vi "FT10_FPGA_7854R_Main 4.vi"(8 "Conn2 DIOs In":T1, 9 "Conn1 DIOs In":T3, 10 "Conn0 DIOs In":T2={"Conn0/DIO_0_7 In"={"Conn0/DIO_0_7 - 75kHz"=FALSE, "Conn0/DIO_0_7 - uSec On"=0, "Conn0/DIO_0_7 In"=[FALSE, FALSE, FALSE, FALSE, FALSE, FALSE, FALSE, FALSE], "Conn0/DIO_0_7 - uSec Off"=0}, "Conn0/DIO_8_15 In"={"Conn0/DIO_8_15 - 75kHz"=FALSE, "Conn0/DIO_8_15 - uSec On"=0, "Conn0/DIO_8_15 In"=[FALSE, FALSE, FALSE, FALSE, FALSE, FALSE, FALSE, FALSE], "Conn0/DIO_8_15 - uSec Off"=0}}, 11 "Connector0/AO0_7":i16[](array[numeric])=[0, 0, 0, 0, 0, 0, 0, 0]) -> (0 "Conn2 - DIOs Out":T4, 1 "Conn1 - DIOs Out":T5, 2 "Conn0 - DIOs Out":T6, 3 "Connector0/AI0":i16[](array[numeric]))   [LabVIEW 2024]
uses:
  <vilib>/rvi/Emulation/niFpgaGetClockAttributes.vi
  <vilib>/rvi/Emulation/niFpgaSctlEmulationGetInTimedLoop.vi
  <vilib>/rvi/Emulation/niFpgaEmulationReportErrorSimple.vi
  <vilib>/rvi/eio/common/nirviEmuTemplateMethod_errors.vi
  <vilib>/rvi/Emulation/niFpgaCriticalErrorInLSC.vi
  <vilib>/eio/EIONode/EIONode.xnode
panel:
  # "Inputs"
  # "Outputs"
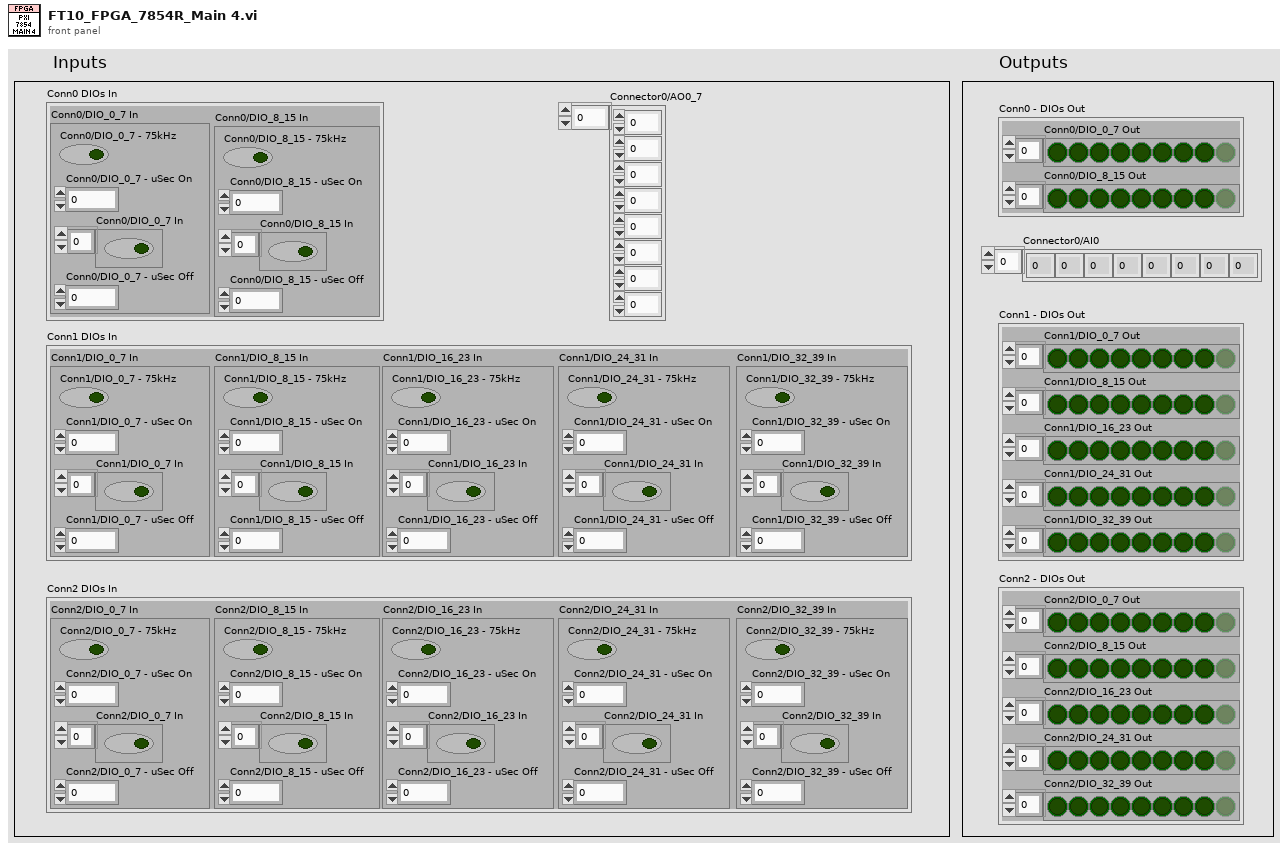
[diagram p1: front panel]
types:
  T1 = cluster{"Conn2/DIO_0_7 In":cluster{"Conn2/DIO_0_7 - 75kHz":bool, "Conn2/DIO_0_7 - uSec On":u16, "Conn2/DIO_0_7 In":bool[], "Conn2/DIO_0_7 - uSec Off":u16}, "Conn2/DIO_8_15 In":cluster{"Conn2/DIO_8_15 - 75kHz":bool, "Conn2/DIO_8_15 - uSec On":u16, "Conn2/DIO_8_15 In":bool[], "Conn2/DIO_8_15 - uSec Off":u16}, "Conn2/DIO_16_23 In":cluster{"Conn2/DIO_16_23 - 75kHz":bool, "Conn2/DIO_16_23 - uSec On":u16, "Conn2/DIO_16_23 In":bool[], "Conn2/DIO_16_23 - uSec Off":u16}, "Conn2/DIO_24_31 In":cluster{"Conn2/DIO_24_31 - 75kHz":bool, "Conn2/DIO_24_31 - uSec On":u16, "Conn2/DIO_24_31 In":bool[], "Conn2/DIO_24_31 - uSec Off":u16}, "Conn2/DIO_32_39 In":cluster{"Conn2/DIO_32_39 - 75kHz":bool, "Conn2/DIO_32_39 - uSec On":u16, "Conn2/DIO_32_39 In":bool[], "Conn2/DIO_32_39 - uSec Off":u16}}
  T2 = cluster{"Conn0/DIO_0_7 In":cluster{"Conn0/DIO_0_7 - 75kHz":bool, "Conn0/DIO_0_7 - uSec On":u16, "Conn0/DIO_0_7 In":bool[], "Conn0/DIO_0_7 - uSec Off":u16}, "Conn0/DIO_8_15 In":cluster{"Conn0/DIO_8_15 - 75kHz":bool, "Conn0/DIO_8_15 - uSec On":u16, "Conn0/DIO_8_15 In":bool[], "Conn0/DIO_8_15 - uSec Off":u16}}
  T3 = cluster{"Conn1/DIO_0_7 In":cluster{"Conn1/DIO_0_7 - 75kHz":bool, "Conn1/DIO_0_7 - uSec On":u16, "Conn1/DIO_0_7 In":bool[], "Conn1/DIO_0_7 - uSec Off":u16}, "Conn1/DIO_8_15 In":cluster{"Conn1/DIO_8_15 - 75kHz":bool, "Conn1/DIO_8_15 - uSec On":u16, "Conn1/DIO_8_15 In":bool[], "Conn1/DIO_8_15 - uSec Off":u16}, "Conn1/DIO_16_23 In":cluster{"Conn1/DIO_16_23 - 75kHz":bool, "Conn1/DIO_16_23 - uSec On":u16, "Conn1/DIO_16_23 In":bool[], "Conn1/DIO_16_23 - uSec Off":u16}, "Conn1/DIO_24_31 In":cluster{"Conn1/DIO_24_31 - 75kHz":bool, "Conn1/DIO_24_31 - uSec On":u16, "Conn1/DIO_24_31 In":bool[], "Conn1/DIO_24_31 - uSec Off":u16}, "Conn1/DIO_32_39 In":cluster{"Conn1/DIO_32_39 - 75kHz":bool, "Conn1/DIO_32_39 - uSec On":u16, "Conn1/DIO_32_39 In":bool[], "Conn1/DIO_32_39 - uSec Off":u16}}
  T4 = cluster{"Conn2/DIO_0_7 Out":bool[], "Conn2/DIO_8_15 Out":bool[], "Conn2/DIO_16_23 Out":bool[], "Conn2/DIO_24_31 Out":bool[], "Conn2/DIO_32_39 Out":bool[]}
  T5 = cluster{"Conn1/DIO_0_7 Out":bool[], "Conn1/DIO_8_15 Out":bool[], "Conn1/DIO_16_23 Out":bool[], "Conn1/DIO_24_31 Out":bool[], "Conn1/DIO_32_39 Out":bool[]}
  T6 = cluster{"Conn0/DIO_0_7 Out":bool[], "Conn0/DIO_8_15 Out":bool[]}
  T7 = cluster{"Conn0/DIO_0_7 - 75kHz":bool, "Conn0/DIO_0_7 - uSec On":u16, "Conn0/DIO_0_7 In":bool[], "Conn0/DIO_0_7 - uSec Off":u16}
  T8 = cluster{"Conn0/DIO_8_15 - 75kHz":bool, "Conn0/DIO_8_15 - uSec On":u16, "Conn0/DIO_8_15 In":bool[], "Conn0/DIO_8_15 - uSec Off":u16}
  T9 = cluster{"Conn1/DIO_0_7 - 75kHz":bool, "Conn1/DIO_0_7 - uSec On":u16, "Conn1/DIO_0_7 In":bool[], "Conn1/DIO_0_7 - uSec Off":u16}
  T10 = cluster{"Conn1/DIO_8_15 - 75kHz":bool, "Conn1/DIO_8_15 - uSec On":u16, "Conn1/DIO_8_15 In":bool[], "Conn1/DIO_8_15 - uSec Off":u16}
  T11 = cluster{"Conn1/DIO_16_23 - 75kHz":bool, "Conn1/DIO_16_23 - uSec On":u16, "Conn1/DIO_16_23 In":bool[], "Conn1/DIO_16_23 - uSec Off":u16}
  T12 = cluster{"Conn1/DIO_24_31 - 75kHz":bool, "Conn1/DIO_24_31 - uSec On":u16, "Conn1/DIO_24_31 In":bool[], "Conn1/DIO_24_31 - uSec Off":u16}
  T13 = cluster{"Conn1/DIO_32_39 - 75kHz":bool, "Conn1/DIO_32_39 - uSec On":u16, "Conn1/DIO_32_39 In":bool[], "Conn1/DIO_32_39 - uSec Off":u16}
  T14 = cluster{"Conn2/DIO_0_7 - 75kHz":bool, "Conn2/DIO_0_7 - uSec On":u16, "Conn2/DIO_0_7 In":bool[], "Conn2/DIO_0_7 - uSec Off":u16}
  T15 = cluster{"Conn2/DIO_8_15 - 75kHz":bool, "Conn2/DIO_8_15 - uSec On":u16, "Conn2/DIO_8_15 In":bool[], "Conn2/DIO_8_15 - uSec Off":u16}
  T16 = cluster{"Conn2/DIO_16_23 - 75kHz":bool, "Conn2/DIO_16_23 - uSec On":u16, "Conn2/DIO_16_23 In":bool[], "Conn2/DIO_16_23 - uSec Off":u16}
  T17 = cluster{"Conn2/DIO_24_31 - 75kHz":bool, "Conn2/DIO_24_31 - uSec On":u16, "Conn2/DIO_24_31 In":bool[], "Conn2/DIO_24_31 - uSec Off":u16}
  T18 = cluster{"Conn2/DIO_32_39 - 75kHz":bool, "Conn2/DIO_32_39 - uSec On":u16, "Conn2/DIO_32_39 In":bool[], "Conn2/DIO_32_39 - uSec Off":u16}
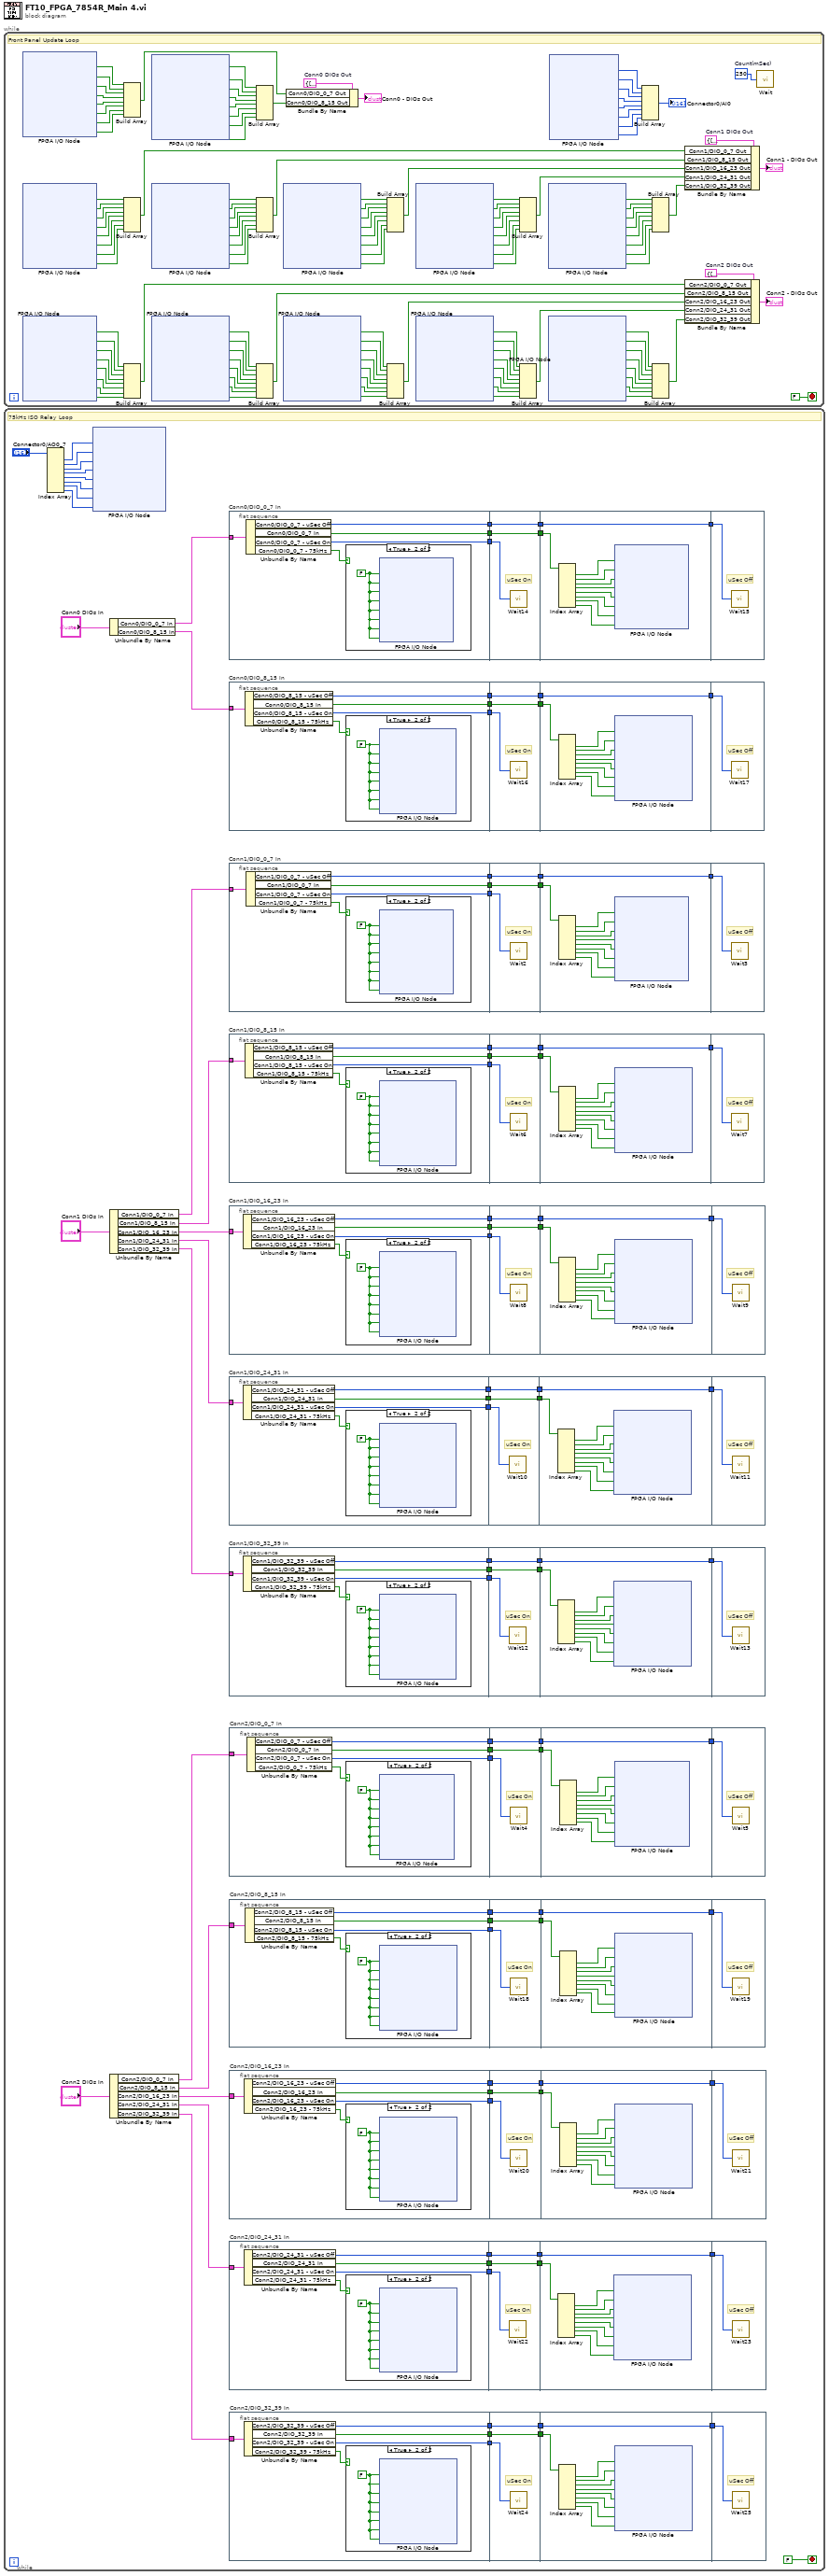
[diagram p0: block diagram]
diagram:
  n1 = while {
    stop <- FALSE stop-if-true
    w16 = T4 {"Conn2/DIO_0_7 Out"=[FALSE, FALSE, FALSE, FALSE, FALSE, FALSE, FALSE, FALSE], "Conn2/DIO_8_15 Out"=[FALSE, FALSE, FALSE, FALSE, FALSE, FALSE, FALSE, FALSE], "Conn2/DIO_16_23 Out"=[FALSE, FALSE, FALSE, FALSE, FALSE, FALSE, FALSE, FALSE], "Conn2/DIO_24_31 Out"=[FALSE, FALSE, FALSE, FALSE, FALSE, FALSE, FALSE, FALSE], "Conn2/DIO_32_39 Out"=[FALSE, FALSE, FALSE, FALSE, FALSE, FALSE, FALSE, FALSE]}  # Conn2 DIOs Out
    w23 = T5 {"Conn1/DIO_0_7 Out"=[FALSE, FALSE, FALSE, FALSE, FALSE, FALSE, FALSE, FALSE], "Conn1/DIO_8_15 Out"=[FALSE, FALSE, FALSE, FALSE, FALSE, FALSE, FALSE, FALSE], "Conn1/DIO_16_23 Out"=[FALSE, FALSE, FALSE, FALSE, FALSE, FALSE, FALSE, FALSE], "Conn1/DIO_24_31 Out"=[FALSE, FALSE, FALSE, FALSE, FALSE, FALSE, FALSE, FALSE], "Conn1/DIO_32_39 Out"=[FALSE, FALSE, FALSE, FALSE, FALSE, FALSE, FALSE, FALSE]}  # Conn1 DIOs Out
    w27 = T6 {"Conn0/DIO_0_7 Out"=[FALSE, FALSE, FALSE, FALSE, FALSE, FALSE, FALSE, FALSE], "Conn0/DIO_8_15 Out"=[FALSE, FALSE, FALSE, FALSE, FALSE, FALSE, FALSE, FALSE]}  # Conn0 DIOs Out
    w124 = u8 250  # Count(mSec)
    # "Front Panel Update Loop"
    n2 = xnode "FPGA I/O Node"() -> ("Connector0/DIO0"=w67:bool, "Connector0/DIO1"=w66:bool, "Connector0/DIO2"=w65:bool, "Connector0/DIO3"=w63:bool, "Connector0/DIO4"=w36:bool, "Connector0/DIO5"=w62:bool, "Connector0/DIO6"=w61:bool, "Connector0/DIO7"=w64:bool)  [unwired: 8 in, 8 out]
    n3 = xnode "FPGA I/O Node"() -> ("Connector1/DIO0"=w107:bool, "Connector1/DIO1"=w106:bool, "Connector1/DIO2"=w105:bool, "Connector1/DIO3"=w104:bool, "Connector1/DIO4"=w103:bool, "Connector1/DIO5"=w102:bool, "Connector1/DIO6"=w101:bool, "Connector1/DIO7"=w100:bool)  [unwired: 8 in, 8 out]
    n4 = xnode "FPGA I/O Node"() -> ("Connector2/DIO0"=w123:bool, "Connector2/DIO1"=w122:bool, "Connector2/DIO2"=w121:bool, "Connector2/DIO3"=w108:bool, "Connector2/DIO4"=w120:bool, "Connector2/DIO5"=w119:bool, "Connector2/DIO6"=w118:bool, "Connector2/DIO7"=w117:bool)  [unwired: 8 in, 8 out]
    n5 = Build Array(w67, w66, w65, w63, w36, w62, w61, w64) -> (w26:bool[])
    n6 = Build Array(w107, w106, w105, w104, w103, w102, w101, w100) -> (w21:bool[])
    n7 = Build Array(w123, w122, w121, w108, w120, w119, w118, w117) -> (w14:bool[])
    n8 = xnode "FPGA I/O Node"() -> ("Connector0/DIO8"=w35:bool, "Connector0/DIO9"=w34:bool, "Connector0/DIO10"=w33:bool, "Connector0/DIO11"=w31:bool, "Connector0/DIO12"=w28:bool, "Connector0/DIO13"=w30:bool, "Connector0/DIO14"=w29:bool, "Connector0/DIO15"=w32:bool)  [unwired: 8 in, 8 out]
    n9 = xnode "FPGA I/O Node"() -> ("Connector1/DIO8"=w93:bool, "Connector1/DIO9"=w95:bool, "Connector1/DIO10"=w94:bool, "Connector1/DIO11"=w92:bool, "Connector1/DIO12"=w91:bool, "Connector1/DIO13"=w90:bool, "Connector1/DIO14"=w89:bool, "Connector1/DIO15"=w88:bool)  [unwired: 8 in, 8 out]
    n10 = xnode "FPGA I/O Node"() -> ("Connector2/DIO8"=w116:bool, "Connector2/DIO9"=w115:bool, "Connector2/DIO10"=w114:bool, "Connector2/DIO11"=w99:bool, "Connector2/DIO12"=w98:bool, "Connector2/DIO13"=w97:bool, "Connector2/DIO14"=w96:bool, "Connector2/DIO15"=w113:bool)  [unwired: 8 in, 8 out]
    n11 = Build Array(w35, w34, w33, w31, w28, w30, w29, w32) -> (w25:bool[])
    n12 = Build Array(w93, w95, w94, w92, w91, w90, w89, w88) -> (w20:bool[])
    n13 = Build Array(w116, w115, w114, w99, w98, w97, w96, w113) -> (w13:bool[])
    n14 = xnode "FPGA I/O Node"() -> ("Connector1/DIO16"=w83:bool, "Connector1/DIO17"=w82:bool, "Connector1/DIO18"=w81:bool, "Connector1/DIO19"=w80:bool, "Connector1/DIO20"=w79:bool, "Connector1/DIO21"=w78:bool, "Connector1/DIO22"=w77:bool, "Connector1/DIO23"=w76:bool)  [unwired: 8 in, 8 out]
    n15 = xnode "FPGA I/O Node"() -> ("Connector2/DIO16"=w112:bool, "Connector2/DIO17"=w111:bool, "Connector2/DIO18"=w110:bool, "Connector2/DIO19"=w87:bool, "Connector2/DIO20"=w86:bool, "Connector2/DIO21"=w85:bool, "Connector2/DIO22"=w84:bool, "Connector2/DIO23"=w109:bool)  [unwired: 8 in, 8 out]
    n16 = Bundle By Name(cluster=w27, "Conn0/DIO_0_7 Out"=w26, "Conn0/DIO_8_15 Out"=w25) -> (→"Conn0 - DIOs Out":T6)
    n17 = Build Array(w83, w82, w81, w80, w79, w78, w77, w76) -> (w19:bool[])
    n18 = Build Array(w112, w111, w110, w87, w86, w85, w84, w109) -> (w12:bool[])
    n19 = xnode "FPGA I/O Node"() -> ("Connector1/DIO24"=w52:bool, "Connector1/DIO25"=w51:bool, "Connector1/DIO26"=w50:bool, "Connector1/DIO27"=w49:bool, "Connector1/DIO28"=w48:bool, "Connector1/DIO29"=w47:bool, "Connector1/DIO30"=w46:bool, "Connector1/DIO31"=w45:bool)  [unwired: 8 in, 8 out]
    n20 = xnode "FPGA I/O Node"() -> ("Connector2/DIO24"=w75:bool, "Connector2/DIO25"=w74:bool, "Connector2/DIO26"=w73:bool, "Connector2/DIO27"=w71:bool, "Connector2/DIO28"=w70:bool, "Connector2/DIO29"=w69:bool, "Connector2/DIO30"=w68:bool, "Connector2/DIO31"=w72:bool)  [unwired: 8 in, 8 out]
    n21 = Build Array(w52, w51, w50, w49, w48, w47, w46, w45) -> (w18:bool[])
    n22 = Build Array(w75, w74, w73, w71, w70, w69, w68, w72) -> (w11:bool[])
    n23 = xnode "FPGA I/O Node"() -> ("Connector1/DIO32"=w44:bool, "Connector1/DIO33"=w43:bool, "Connector1/DIO34"=w42:bool, "Connector1/DIO35"=w41:bool, "Connector1/DIO36"=w40:bool, "Connector1/DIO37"=w39:bool, "Connector1/DIO38"=w38:bool, "Connector1/DIO39"=w37:bool)  [unwired: 8 in, 8 out]
    n24 = xnode "FPGA I/O Node"() -> ("Connector2/DIO32"=w60:bool, "Connector2/DIO33"=w59:bool, "Connector2/DIO34"=w58:bool, "Connector2/DIO35"=w56:bool, "Connector2/DIO36"=w55:bool, "Connector2/DIO37"=w54:bool, "Connector2/DIO38"=w53:bool, "Connector2/DIO39"=w57:bool)  [unwired: 8 in, 8 out]
    n25 = xnode "FPGA I/O Node"() -> ("Connector0/AI0"=w9:i16, "Connector0/AI1"=w8:i16, "Connector0/AI2"=w7:i16, "Connector0/AI3"=w6:i16, "Connector0/AI4"=w2:i16, "Connector0/AI5"=w3:i16, "Connector0/AI6"=w4:i16, "Connector0/AI7"=w5:i16)  [unwired: 8 in, 8 out]
    n26 = Build Array(w9, w8, w7, w6, w2, w3, w4, w5) -> (→"Connector0/AI0":i16[])
    n27 = Build Array(w44, w43, w42, w41, w40, w39, w38, w37) -> (w17:bool[])
    n28 = Build Array(w60, w59, w58, w56, w55, w54, w53, w57) -> (w10:bool[])
    n29 = Bundle By Name(cluster=w23, "Conn1/DIO_0_7 Out"=w21, "Conn1/DIO_8_15 Out"=w20, "Conn1/DIO_16_23 Out"=w19, "Conn1/DIO_24_31 Out"=w18, "Conn1/DIO_32_39 Out"=w17) -> (→"Conn1 - DIOs Out":T5)
    n30 = Bundle By Name(cluster=w16, "Conn2/DIO_0_7 Out"=w14, "Conn2/DIO_8_15 Out"=w13, "Conn2/DIO_16_23 Out"=w12, "Conn2/DIO_24_31 Out"=w11, "Conn2/DIO_32_39 Out"=w10) -> (→"Conn2 - DIOs Out":T4)
    n31 = call "Wait"("Count(mSec)"=w124) -> ()  [unwired: 1 out]
  }
  n32 = while {
    stop <- FALSE stop-if-true
    # "75kHz ISO Relay Loop"
    n33 = Index Array(array="Connector0/AO0_7") -> (element #1=w169:i16, element #2=w168:i16, element #3=w167:i16, element #4=w163:i16, element #5=w162:i16, element #6=w164:i16, element #7=w165:i16, element #8=w166:i16)  [unwired: 8 in]
    n34 = xnode "FPGA I/O Node"("Connector0/AO0"=w169, "Connector0/AO1"=w168, "Connector0/AO2"=w167, "Connector0/AO3"=w163, "Connector0/AO4"=w162, "Connector0/AO5"=w164, "Connector0/AO6"=w165, "Connector0/AO7"=w166) -> ()  [unwired: 8 in, 8 out]
    n35 = Unbundle By Name("Conn0 DIOs In") -> ("Conn0/DIO_0_7 In"=w172:T7, "Conn0/DIO_8_15 In"=w171:T8)
    n36 = Unbundle By Name("Conn1 DIOs In") -> ("Conn1/DIO_0_7 In"=w214:T9, "Conn1/DIO_8_15 In"=w188:T10, "Conn1/DIO_16_23 In"=w186:T11, "Conn1/DIO_24_31 In"=w187:T12, "Conn1/DIO_32_39 In"=w189:T13)
    n37 = Unbundle By Name("Conn2 DIOs In") -> ("Conn2/DIO_0_7 In"=w129:T14, "Conn2/DIO_8_15 In"=w128:T15, "Conn2/DIO_16_23 In"=w130:T16, "Conn2/DIO_24_31 In"=w127:T17, "Conn2/DIO_32_39 In"=w126:T18)
    n38 = flat-sequence "Conn0/DIO_0_7 In" {
      tunnel: [w346] -> w185
      tunnel: [w345] -> w184
      tunnel: [w344] -> w183
      tunnel: w172 -> [w343]
      tunnel: w185 -> [w351]
      tunnel: w184 -> [w350]
      tunnel: w183 -> [w349]
      tunnel: [w350] -> w182
      tunnel: [w349] -> w181
      tunnel: w182 -> [w353]
      tunnel: [w352] -> w180
      tunnel: w181 -> [w352]
      tunnel: w180 -> [w362]
      frame #0 {
        n39 = Unbundle By Name(w343) -> ("Conn0/DIO_0_7 - uSec Off"=w344:u16, "Conn0/DIO_0_7 In"=w345:bool[], "Conn0/DIO_0_7 - uSec On"=w346:u16, "Conn0/DIO_0_7 - 75kHz"=w347:bool)
        n40 = case shown="True" w347 {
          frame False {
          }
          frame True {
            w348 = FALSE ("Connector1/DIO0")
            n41 = xnode "FPGA I/O Node"("Connector0/DIO0"=w348, "Connector0/DIO1"=w348, "Connector0/DIO2"=w348, "Connector0/DIO3"=w348, "Connector0/DIO4"=w348, "Connector0/DIO5"=w348, "Connector0/DIO6"=w348, "Connector0/DIO7"=w348) -> ()  [unwired: 8 in, 8 out]
          }
        }
      }
      frame #1 {
        # "uSec On"
        n42 = call "Wait14"("Count(uSec)"=w351) -> ()  [unwired: 1 out]
      }
      frame #2 {
        n43 = Index Array(array=w353) -> (element #1=w355:bool, element #2=w356:bool, element #3=w357:bool, element #4=w358:bool, element #5=w359:bool, element #6=w360:bool, element #7=w361:bool, element #8=w354:bool)  [unwired: 8 in]
        n44 = xnode "FPGA I/O Node"("Connector0/DIO0"=w355, "Connector0/DIO1"=w356, "Connector0/DIO2"=w357, "Connector0/DIO3"=w358, "Connector0/DIO4"=w359, "Connector0/DIO5"=w360, "Connector0/DIO6"=w361, "Connector0/DIO7"=w354) -> ()  [unwired: 8 in, 8 out]
      }
      frame #3 {
        # "uSec Off"
        n45 = call "Wait15"("Count(uSec)"=w362) -> ()  [unwired: 1 out]
      }
    }
    n46 = flat-sequence "Conn0/DIO_8_15 In" {
      tunnel: [w326] -> w179
      tunnel: [w325] -> w178
      tunnel: [w324] -> w177
      tunnel: w171 -> [w323]
      tunnel: w179 -> [w331]
      tunnel: w178 -> [w330]
      tunnel: w177 -> [w329]
      tunnel: [w330] -> w176
      tunnel: [w329] -> w175
      tunnel: w176 -> [w333]
      tunnel: [w332] -> w174
      tunnel: w175 -> [w332]
      tunnel: w174 -> [w342]
      frame #0 {
        n47 = Unbundle By Name(w323) -> ("Conn0/DIO_8_15 - uSec Off"=w324:u16, "Conn0/DIO_8_15 In"=w325:bool[], "Conn0/DIO_8_15 - uSec On"=w326:u16, "Conn0/DIO_8_15 - 75kHz"=w327:bool)
        n48 = case shown="True" w327 {
          frame False {
          }
          frame True {
            w328 = FALSE ("Connector1/DIO0")
            n49 = xnode "FPGA I/O Node"("Connector0/DIO8"=w328, "Connector0/DIO9"=w328, "Connector0/DIO10"=w328, "Connector0/DIO11"=w328, "Connector0/DIO12"=w328, "Connector0/DIO13"=w328, "Connector0/DIO14"=w328, "Connector0/DIO15"=w328) -> ()  [unwired: 8 in, 8 out]
          }
        }
      }
      frame #1 {
        # "uSec On"
        n50 = call "Wait16"("Count(uSec)"=w331) -> ()  [unwired: 1 out]
      }
      frame #2 {
        n51 = Index Array(array=w333) -> (element #1=w335:bool, element #2=w336:bool, element #3=w337:bool, element #4=w338:bool, element #5=w339:bool, element #6=w340:bool, element #7=w341:bool, element #8=w334:bool)  [unwired: 8 in]
        n52 = xnode "FPGA I/O Node"("Connector0/DIO8"=w335, "Connector0/DIO9"=w336, "Connector0/DIO10"=w337, "Connector0/DIO11"=w338, "Connector0/DIO12"=w339, "Connector0/DIO13"=w340, "Connector0/DIO14"=w341, "Connector0/DIO15"=w334) -> ()  [unwired: 8 in, 8 out]
      }
      frame #3 {
        # "uSec Off"
        n53 = call "Wait17"("Count(uSec)"=w342) -> ()  [unwired: 1 out]
      }
    }
    n54 = flat-sequence "Conn1/DIO_0_7 In" {
      tunnel: [w446] -> w221
      tunnel: [w445] -> w220
      tunnel: [w444] -> w219
      tunnel: w214 -> [w443]
      tunnel: w221 -> [w451]
      tunnel: w220 -> [w450]
      tunnel: w219 -> [w449]
      tunnel: [w450] -> w218
      tunnel: [w449] -> w216
      tunnel: w218 -> [w453]
      tunnel: [w452] -> w217
      tunnel: w216 -> [w452]
      tunnel: w217 -> [w462]
      frame #0 {
        n55 = Unbundle By Name(w443) -> ("Conn1/DIO_0_7 - uSec Off"=w444:u16, "Conn1/DIO_0_7 In"=w445:bool[], "Conn1/DIO_0_7 - uSec On"=w446:u16, "Conn1/DIO_0_7 - 75kHz"=w447:bool)
        n56 = case shown="True" w447 {
          frame False {
          }
          frame True {
            w448 = FALSE ("Connector1/DIO0")
            n57 = xnode "FPGA I/O Node"("Connector1/DIO0"=w448, "Connector1/DIO1"=w448, "Connector1/DIO2"=w448, "Connector1/DIO3"=w448, "Connector1/DIO4"=w448, "Connector1/DIO5"=w448, "Connector1/DIO6"=w448, "Connector1/DIO7"=w448) -> ()  [unwired: 8 in, 8 out]
          }
        }
      }
      frame #1 {
        # "uSec On"
        n58 = call "Wait2"("Count(uSec)"=w451) -> ()  [unwired: 1 out]
      }
      frame #2 {
        n59 = Index Array(array=w453) -> (element #1=w455:bool, element #2=w456:bool, element #3=w457:bool, element #4=w458:bool, element #5=w459:bool, element #6=w460:bool, element #7=w461:bool, element #8=w454:bool)  [unwired: 8 in]
        n60 = xnode "FPGA I/O Node"("Connector1/DIO0"=w455, "Connector1/DIO1"=w456, "Connector1/DIO2"=w457, "Connector1/DIO3"=w458, "Connector1/DIO4"=w459, "Connector1/DIO5"=w460, "Connector1/DIO6"=w461, "Connector1/DIO7"=w454) -> ()  [unwired: 8 in, 8 out]
      }
      frame #3 {
        # "uSec Off"
        n61 = call "Wait3"("Count(uSec)"=w462) -> ()  [unwired: 1 out]
      }
    }
    n62 = flat-sequence "Conn1/DIO_8_15 In" {
      tunnel: [w426] -> w213
      tunnel: [w425] -> w212
      tunnel: [w424] -> w211
      tunnel: w188 -> [w423]
      tunnel: w213 -> [w431]
      tunnel: w212 -> [w430]
      tunnel: w211 -> [w429]
      tunnel: [w430] -> w210
      tunnel: [w429] -> w209
      tunnel: w210 -> [w433]
      tunnel: [w432] -> w208
      tunnel: w209 -> [w432]
      tunnel: w208 -> [w442]
      frame #0 {
        n63 = Unbundle By Name(w423) -> ("Conn1/DIO_8_15 - uSec Off"=w424:u16, "Conn1/DIO_8_15 In"=w425:bool[], "Conn1/DIO_8_15 - uSec On"=w426:u16, "Conn1/DIO_8_15 - 75kHz"=w427:bool)
        n64 = case shown="True" w427 {
          frame False {
          }
          frame True {
            w428 = FALSE ("Connector1/DIO0")
            n65 = xnode "FPGA I/O Node"("Connector1/DIO8"=w428, "Connector1/DIO9"=w428, "Connector1/DIO10"=w428, "Connector1/DIO11"=w428, "Connector1/DIO12"=w428, "Connector1/DIO13"=w428, "Connector1/DIO14"=w428, "Connector1/DIO15"=w428) -> ()  [unwired: 8 in, 8 out]
          }
        }
      }
      frame #1 {
        # "uSec On"
        n66 = call "Wait6"("Count(uSec)"=w431) -> ()  [unwired: 1 out]
      }
      frame #2 {
        n67 = Index Array(array=w433) -> (element #1=w435:bool, element #2=w436:bool, element #3=w437:bool, element #4=w438:bool, element #5=w439:bool, element #6=w440:bool, element #7=w441:bool, element #8=w434:bool)  [unwired: 8 in]
        n68 = xnode "FPGA I/O Node"("Connector1/DIO8"=w435, "Connector1/DIO9"=w436, "Connector1/DIO10"=w437, "Connector1/DIO11"=w438, "Connector1/DIO12"=w439, "Connector1/DIO13"=w440, "Connector1/DIO14"=w441, "Connector1/DIO15"=w434) -> ()  [unwired: 8 in, 8 out]
      }
      frame #3 {
        # "uSec Off"
        n69 = call "Wait7"("Count(uSec)"=w442) -> ()  [unwired: 1 out]
      }
    }
    n70 = flat-sequence "Conn1/DIO_16_23 In" {
      tunnel: [w406] -> w207
      tunnel: [w405] -> w206
      tunnel: [w404] -> w205
      tunnel: w186 -> [w403]
      tunnel: w207 -> [w411]
      tunnel: w206 -> [w410]
      tunnel: w205 -> [w409]
      tunnel: [w410] -> w204
      tunnel: [w409] -> w203
      tunnel: w204 -> [w413]
      tunnel: [w412] -> w202
      tunnel: w203 -> [w412]
      tunnel: w202 -> [w422]
      frame #0 {
        n71 = Unbundle By Name(w403) -> ("Conn1/DIO_16_23 - uSec Off"=w404:u16, "Conn1/DIO_16_23 In"=w405:bool[], "Conn1/DIO_16_23 - uSec On"=w406:u16, "Conn1/DIO_16_23 - 75kHz"=w407:bool)
        n72 = case shown="True" w407 {
          frame False {
          }
          frame True {
            w408 = FALSE ("Connector1/DIO0")
            n73 = xnode "FPGA I/O Node"("Connector1/DIO16"=w408, "Connector1/DIO17"=w408, "Connector1/DIO18"=w408, "Connector1/DIO19"=w408, "Connector1/DIO20"=w408, "Connector1/DIO21"=w408, "Connector1/DIO22"=w408, "Connector1/DIO23"=w408) -> ()  [unwired: 8 in, 8 out]
          }
        }
      }
      frame #1 {
        # "uSec On"
        n74 = call "Wait8"("Count(uSec)"=w411) -> ()  [unwired: 1 out]
      }
      frame #2 {
        n75 = Index Array(array=w413) -> (element #1=w415:bool, element #2=w416:bool, element #3=w417:bool, element #4=w418:bool, element #5=w419:bool, element #6=w420:bool, element #7=w421:bool, element #8=w414:bool)  [unwired: 8 in]
        n76 = xnode "FPGA I/O Node"("Connector1/DIO16"=w415, "Connector1/DIO17"=w416, "Connector1/DIO18"=w417, "Connector1/DIO19"=w418, "Connector1/DIO20"=w419, "Connector1/DIO21"=w420, "Connector1/DIO22"=w421, "Connector1/DIO23"=w414) -> ()  [unwired: 8 in, 8 out]
      }
      frame #3 {
        # "uSec Off"
        n77 = call "Wait9"("Count(uSec)"=w422) -> ()  [unwired: 1 out]
      }
    }
    n78 = flat-sequence "Conn1/DIO_24_31 In" {
      tunnel: [w386] -> w201
      tunnel: [w385] -> w200
      tunnel: [w384] -> w199
      tunnel: w187 -> [w383]
      tunnel: w201 -> [w391]
      tunnel: w200 -> [w390]
      tunnel: w199 -> [w389]
      tunnel: [w390] -> w198
      tunnel: [w389] -> w197
      tunnel: w198 -> [w393]
      tunnel: [w392] -> w196
      tunnel: w197 -> [w392]
      tunnel: w196 -> [w402]
      frame #0 {
        n79 = Unbundle By Name(w383) -> ("Conn1/DIO_24_31 - uSec Off"=w384:u16, "Conn1/DIO_24_31 In"=w385:bool[], "Conn1/DIO_24_31 - uSec On"=w386:u16, "Conn1/DIO_24_31 - 75kHz"=w387:bool)
        n80 = case shown="True" w387 {
          frame False {
          }
          frame True {
            w388 = FALSE ("Connector1/DIO0")
            n81 = xnode "FPGA I/O Node"("Connector1/DIO24"=w388, "Connector1/DIO25"=w388, "Connector1/DIO26"=w388, "Connector1/DIO27"=w388, "Connector1/DIO28"=w388, "Connector1/DIO29"=w388, "Connector1/DIO30"=w388, "Connector1/DIO31"=w388) -> ()  [unwired: 8 in, 8 out]
          }
        }
      }
      frame #1 {
        # "uSec On"
        n82 = call "Wait10"("Count(uSec)"=w391) -> ()  [unwired: 1 out]
      }
      frame #2 {
        n83 = Index Array(array=w393) -> (element #1=w395:bool, element #2=w396:bool, element #3=w397:bool, element #4=w398:bool, element #5=w399:bool, element #6=w400:bool, element #7=w401:bool, element #8=w394:bool)  [unwired: 8 in]
        n84 = xnode "FPGA I/O Node"("Connector1/DIO24"=w395, "Connector1/DIO25"=w396, "Connector1/DIO26"=w397, "Connector1/DIO27"=w398, "Connector1/DIO28"=w399, "Connector1/DIO29"=w400, "Connector1/DIO30"=w401, "Connector1/DIO31"=w394) -> ()  [unwired: 8 in, 8 out]
      }
      frame #3 {
        # "uSec Off"
        n85 = call "Wait11"("Count(uSec)"=w402) -> ()  [unwired: 1 out]
      }
    }
    n86 = flat-sequence "Conn1/DIO_32_39 In" {
      tunnel: [w366] -> w195
      tunnel: [w365] -> w194
      tunnel: [w364] -> w193
      tunnel: w189 -> [w363]
      tunnel: w195 -> [w371]
      tunnel: w194 -> [w370]
      tunnel: w193 -> [w369]
      tunnel: [w370] -> w192
      tunnel: [w369] -> w191
      tunnel: w192 -> [w373]
      tunnel: [w372] -> w190
      tunnel: w191 -> [w372]
      tunnel: w190 -> [w382]
      frame #0 {
        n87 = Unbundle By Name(w363) -> ("Conn1/DIO_32_39 - uSec Off"=w364:u16, "Conn1/DIO_32_39 In"=w365:bool[], "Conn1/DIO_32_39 - uSec On"=w366:u16, "Conn1/DIO_32_39 - 75kHz"=w367:bool)
        n88 = case shown="True" w367 {
          frame False {
          }
          frame True {
            w368 = FALSE ("Connector1/DIO0")
            n89 = xnode "FPGA I/O Node"("Connector1/DIO32"=w368, "Connector1/DIO33"=w368, "Connector1/DIO34"=w368, "Connector1/DIO35"=w368, "Connector1/DIO36"=w368, "Connector1/DIO37"=w368, "Connector1/DIO38"=w368, "Connector1/DIO39"=w368) -> ()  [unwired: 8 in, 8 out]
          }
        }
      }
      frame #1 {
        # "uSec On"
        n90 = call "Wait12"("Count(uSec)"=w371) -> ()  [unwired: 1 out]
      }
      frame #2 {
        n91 = Index Array(array=w373) -> (element #1=w375:bool, element #2=w376:bool, element #3=w377:bool, element #4=w378:bool, element #5=w379:bool, element #6=w380:bool, element #7=w381:bool, element #8=w374:bool)  [unwired: 8 in]
        n92 = xnode "FPGA I/O Node"("Connector1/DIO32"=w375, "Connector1/DIO33"=w376, "Connector1/DIO34"=w377, "Connector1/DIO35"=w378, "Connector1/DIO36"=w379, "Connector1/DIO37"=w380, "Connector1/DIO38"=w381, "Connector1/DIO39"=w374) -> ()  [unwired: 8 in, 8 out]
      }
      frame #3 {
        # "uSec Off"
        n93 = call "Wait13"("Count(uSec)"=w382) -> ()  [unwired: 1 out]
      }
    }
    n94 = flat-sequence "Conn2/DIO_0_7 In" {
      tunnel: [w306] -> w161
      tunnel: [w305] -> w160
      tunnel: [w304] -> w159
      tunnel: w129 -> [w303]
      tunnel: w161 -> [w311]
      tunnel: w160 -> [w310]
      tunnel: w159 -> [w309]
      tunnel: [w310] -> w158
      tunnel: [w309] -> w157
      tunnel: w158 -> [w313]
      tunnel: [w312] -> w156
      tunnel: w157 -> [w312]
      tunnel: w156 -> [w322]
      frame #0 {
        n95 = Unbundle By Name(w303) -> ("Conn2/DIO_0_7 - uSec Off"=w304:u16, "Conn2/DIO_0_7 In"=w305:bool[], "Conn2/DIO_0_7 - uSec On"=w306:u16, "Conn2/DIO_0_7 - 75kHz"=w307:bool)
        n96 = case shown="True" w307 {
          frame False {
          }
          frame True {
            w308 = FALSE ("Connector1/DIO0")
            n97 = xnode "FPGA I/O Node"("Connector2/DIO0"=w308, "Connector2/DIO1"=w308, "Connector2/DIO2"=w308, "Connector2/DIO3"=w308, "Connector2/DIO4"=w308, "Connector2/DIO5"=w308, "Connector2/DIO6"=w308, "Connector2/DIO7"=w308) -> ()  [unwired: 8 in, 8 out]
          }
        }
      }
      frame #1 {
        # "uSec On"
        n98 = call "Wait4"("Count(uSec)"=w311) -> ()  [unwired: 1 out]
      }
      frame #2 {
        n99 = Index Array(array=w313) -> (element #1=w315:bool, element #2=w316:bool, element #3=w317:bool, element #4=w318:bool, element #5=w319:bool, element #6=w320:bool, element #7=w321:bool, element #8=w314:bool)  [unwired: 8 in]
        n100 = xnode "FPGA I/O Node"("Connector2/DIO0"=w315, "Connector2/DIO1"=w316, "Connector2/DIO2"=w317, "Connector2/DIO3"=w318, "Connector2/DIO4"=w319, "Connector2/DIO5"=w320, "Connector2/DIO6"=w321, "Connector2/DIO7"=w314) -> ()  [unwired: 8 in, 8 out]
      }
      frame #3 {
        # "uSec Off"
        n101 = call "Wait5"("Count(uSec)"=w322) -> ()  [unwired: 1 out]
      }
    }
    n102 = flat-sequence "Conn2/DIO_8_15 In" {
      tunnel: [w286] -> w155
      tunnel: [w285] -> w154
      tunnel: [w284] -> w153
      tunnel: w128 -> [w283]
      tunnel: w155 -> [w291]
      tunnel: w154 -> [w290]
      tunnel: w153 -> [w289]
      tunnel: [w290] -> w152
      tunnel: [w289] -> w151
      tunnel: w152 -> [w293]
      tunnel: [w292] -> w150
      tunnel: w151 -> [w292]
      tunnel: w150 -> [w302]
      frame #0 {
        n103 = Unbundle By Name(w283) -> ("Conn2/DIO_8_15 - uSec Off"=w284:u16, "Conn2/DIO_8_15 In"=w285:bool[], "Conn2/DIO_8_15 - uSec On"=w286:u16, "Conn2/DIO_8_15 - 75kHz"=w287:bool)
        n104 = case shown="True" w287 {
          frame False {
          }
          frame True {
            w288 = FALSE ("Connector1/DIO0")
            n105 = xnode "FPGA I/O Node"("Connector2/DIO8"=w288, "Connector2/DIO9"=w288, "Connector2/DIO10"=w288, "Connector2/DIO11"=w288, "Connector2/DIO12"=w288, "Connector2/DIO13"=w288, "Connector2/DIO14"=w288, "Connector2/DIO15"=w288) -> ()  [unwired: 8 in, 8 out]
          }
        }
      }
      frame #1 {
        # "uSec On"
        n106 = call "Wait18"("Count(uSec)"=w291) -> ()  [unwired: 1 out]
      }
      frame #2 {
        n107 = Index Array(array=w293) -> (element #1=w295:bool, element #2=w296:bool, element #3=w297:bool, element #4=w298:bool, element #5=w299:bool, element #6=w300:bool, element #7=w301:bool, element #8=w294:bool)  [unwired: 8 in]
        n108 = xnode "FPGA I/O Node"("Connector2/DIO8"=w295, "Connector2/DIO9"=w296, "Connector2/DIO10"=w297, "Connector2/DIO11"=w298, "Connector2/DIO12"=w299, "Connector2/DIO13"=w300, "Connector2/DIO14"=w301, "Connector2/DIO15"=w294) -> ()  [unwired: 8 in, 8 out]
      }
      frame #3 {
        # "uSec Off"
        n109 = call "Wait19"("Count(uSec)"=w302) -> ()  [unwired: 1 out]
      }
    }
    n110 = flat-sequence "Conn2/DIO_16_23 In" {
      tunnel: [w266] -> w149
      tunnel: [w265] -> w148
      tunnel: [w264] -> w147
      tunnel: w130 -> [w263]
      tunnel: w149 -> [w271]
      tunnel: w148 -> [w270]
      tunnel: w147 -> [w269]
      tunnel: [w270] -> w146
      tunnel: [w269] -> w145
      tunnel: w146 -> [w273]
      tunnel: [w272] -> w144
      tunnel: w145 -> [w272]
      tunnel: w144 -> [w282]
      frame #0 {
        n111 = Unbundle By Name(w263) -> ("Conn2/DIO_16_23 - uSec Off"=w264:u16, "Conn2/DIO_16_23 In"=w265:bool[], "Conn2/DIO_16_23 - uSec On"=w266:u16, "Conn2/DIO_16_23 - 75kHz"=w267:bool)
        n112 = case shown="True" w267 {
          frame False {
          }
          frame True {
            w268 = FALSE ("Connector1/DIO0")
            n113 = xnode "FPGA I/O Node"("Connector2/DIO16"=w268, "Connector2/DIO17"=w268, "Connector2/DIO18"=w268, "Connector2/DIO19"=w268, "Connector2/DIO20"=w268, "Connector2/DIO21"=w268, "Connector2/DIO22"=w268, "Connector2/DIO23"=w268) -> ()  [unwired: 8 in, 8 out]
          }
        }
      }
      frame #1 {
        # "uSec On"
        n114 = call "Wait20"("Count(uSec)"=w271) -> ()  [unwired: 1 out]
      }
      frame #2 {
        n115 = Index Array(array=w273) -> (element #1=w275:bool, element #2=w276:bool, element #3=w277:bool, element #4=w278:bool, element #5=w279:bool, element #6=w280:bool, element #7=w281:bool, element #8=w274:bool)  [unwired: 8 in]
        n116 = xnode "FPGA I/O Node"("Connector2/DIO16"=w275, "Connector2/DIO17"=w276, "Connector2/DIO18"=w277, "Connector2/DIO19"=w278, "Connector2/DIO20"=w279, "Connector2/DIO21"=w280, "Connector2/DIO22"=w281, "Connector2/DIO23"=w274) -> ()  [unwired: 8 in, 8 out]
      }
      frame #3 {
        # "uSec Off"
        n117 = call "Wait21"("Count(uSec)"=w282) -> ()  [unwired: 1 out]
      }
    }
    n118 = flat-sequence "Conn2/DIO_24_31 In" {
      tunnel: [w246] -> w143
      tunnel: [w245] -> w142
      tunnel: [w244] -> w141
      tunnel: w127 -> [w243]
      tunnel: w143 -> [w251]
      tunnel: w142 -> [w250]
      tunnel: w141 -> [w249]
      tunnel: [w250] -> w140
      tunnel: [w249] -> w139
      tunnel: w140 -> [w253]
      tunnel: [w252] -> w138
      tunnel: w139 -> [w252]
      tunnel: w138 -> [w262]
      frame #0 {
        n119 = Unbundle By Name(w243) -> ("Conn2/DIO_24_31 - uSec Off"=w244:u16, "Conn2/DIO_24_31 In"=w245:bool[], "Conn2/DIO_24_31 - uSec On"=w246:u16, "Conn2/DIO_24_31 - 75kHz"=w247:bool)
        n120 = case shown="True" w247 {
          frame False {
          }
          frame True {
            w248 = FALSE ("Connector1/DIO0")
            n121 = xnode "FPGA I/O Node"("Connector2/DIO24"=w248, "Connector2/DIO25"=w248, "Connector2/DIO26"=w248, "Connector2/DIO27"=w248, "Connector2/DIO28"=w248, "Connector2/DIO29"=w248, "Connector2/DIO30"=w248, "Connector2/DIO31"=w248) -> ()  [unwired: 8 in, 8 out]
          }
        }
      }
      frame #1 {
        # "uSec On"
        n122 = call "Wait22"("Count(uSec)"=w251) -> ()  [unwired: 1 out]
      }
      frame #2 {
        n123 = Index Array(array=w253) -> (element #1=w255:bool, element #2=w256:bool, element #3=w257:bool, element #4=w258:bool, element #5=w259:bool, element #6=w260:bool, element #7=w261:bool, element #8=w254:bool)  [unwired: 8 in]
        n124 = xnode "FPGA I/O Node"("Connector2/DIO24"=w255, "Connector2/DIO25"=w256, "Connector2/DIO26"=w257, "Connector2/DIO27"=w258, "Connector2/DIO28"=w259, "Connector2/DIO29"=w260, "Connector2/DIO30"=w261, "Connector2/DIO31"=w254) -> ()  [unwired: 8 in, 8 out]
      }
      frame #3 {
        # "uSec Off"
        n125 = call "Wait23"("Count(uSec)"=w262) -> ()  [unwired: 1 out]
      }
    }
    n126 = flat-sequence "Conn2/DIO_32_39 In" {
      tunnel: [w226] -> w137
      tunnel: [w225] -> w136
      tunnel: [w224] -> w135
      tunnel: w126 -> [w223]
      tunnel: w137 -> [w231]
      tunnel: w136 -> [w230]
      tunnel: w135 -> [w229]
      tunnel: [w230] -> w134
      tunnel: [w229] -> w133
      tunnel: w134 -> [w233]
      tunnel: [w232] -> w132
      tunnel: w133 -> [w232]
      tunnel: w132 -> [w242]
      frame #0 {
        n127 = Unbundle By Name(w223) -> ("Conn2/DIO_32_39 - uSec Off"=w224:u16, "Conn2/DIO_32_39 In"=w225:bool[], "Conn2/DIO_32_39 - uSec On"=w226:u16, "Conn2/DIO_32_39 - 75kHz"=w227:bool)
        n128 = case shown="True" w227 {
          frame False {
          }
          frame True {
            w228 = FALSE ("Connector1/DIO0")
            n129 = xnode "FPGA I/O Node"("Connector2/DIO32"=w228, "Connector2/DIO33"=w228, "Connector2/DIO34"=w228, "Connector2/DIO35"=w228, "Connector2/DIO36"=w228, "Connector2/DIO37"=w228, "Connector2/DIO38"=w228, "Connector2/DIO39"=w228) -> ()  [unwired: 8 in, 8 out]
          }
        }
      }
      frame #1 {
        # "uSec On"
        n130 = call "Wait24"("Count(uSec)"=w231) -> ()  [unwired: 1 out]
      }
      frame #2 {
        n131 = Index Array(array=w233) -> (element #1=w235:bool, element #2=w236:bool, element #3=w237:bool, element #4=w238:bool, element #5=w239:bool, element #6=w240:bool, element #7=w241:bool, element #8=w234:bool)  [unwired: 8 in]
        n132 = xnode "FPGA I/O Node"("Connector2/DIO32"=w235, "Connector2/DIO33"=w236, "Connector2/DIO34"=w237, "Connector2/DIO35"=w238, "Connector2/DIO36"=w239, "Connector2/DIO37"=w240, "Connector2/DIO38"=w241, "Connector2/DIO39"=w234) -> ()  [unwired: 8 in, 8 out]
      }
      frame #3 {
        # "uSec Off"
        n133 = call "Wait25"("Count(uSec)"=w242) -> ()  [unwired: 1 out]
      }
    }
  }
